vi "ROI entry-Previous ROI compat-Zoom.vi"(8 "error in (no error)":errorcluster, 9 "Proceed":bool=TRUE, 11 "Old ROI file path":path) -> (0 "error out":errorcluster, 1 "Proceed":bool, 3 "Old ROI file path (dup)":path)   [LabVIEW 2013]
uses:
  Visualisation/Functional Imaging Viewer/SubVIs/Experiment header interface/Typedefs/Header file type enum.ctl
  Visualisation/Functional Imaging Viewer/SubVIs/Experiment header interface/Typedefs/Save-Load-Save as-Load last enum.ctl
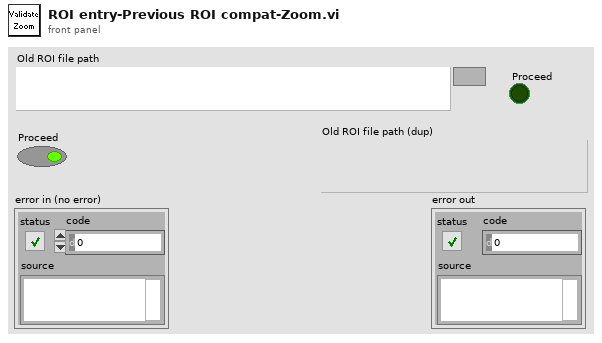
[diagram p1: front panel]
types:
  T1 = typedef "Save-Load-Save as-Load last enum.ctl" = enum16{"Save file", "Save file as", "Load file", "Load last file"}
  T2 = typedef "Header file type enum.ctl" = enum16{"All parameters", "Params for funct acq w ROI or mscn", "Params for funct acq w rectangles", "Live imaging header parameters", "AOL Parameters"}
  T3 = typedef "Fixed strings.ctl" = cluster{"ROI file name":string, "Normalised ROI file name":string, "Zplane Pockels values file name":string, "Functional data folder name":string, "Experiment Header file name":string, "Z-stack images folder name":string, "Groups setup rel. path":string, "Groups text file rel. path":string, "TDMS files folder name (F.img)":string, "TDMS files folder name (V.acq)":string, "TDMS files folder name (Pl.acq)":string, "Cycle rel times sequence file":string, "Dynamically called VIs folder name":string, "Time Series folder base name":string}
  T4 = typedef "Header parameters cluster-ALL.ctl" = cluster{"Imaging Protocol":T5, "Number of POI":u16, "Number of Miniscans":u16, "Number of Trials":u16, "Number of Cycles ":u64, "# Averaged Frames":u16, "Laser power (%)":u8, "Pockels":dbl, "Acquisition Length (sec)":dbl, "Fill time (us)":dbl, "POI Dwell time (us)":dbl, "Miniscan Dwell time per pixel (us)":dbl, "PMT 1":dbl, "PMT 2":dbl, "Back Apperture":dbl, "Zoom":dbl, "Frame Size":T6, "Center Frequency":dbl, "Field of View":dbl, "DwellTime (us)":dbl, "Wavelength (nm)":dbl, "AOL Z":dbl, "AOL Mode":T7, "GridXY":dbl, "GridZ":dbl, "TriggerDelay (sec)":dbl, "Number of Pixels in Miniscan":u16, "Experiment folder path":path, "X centre":dbl, "Y centre":dbl, "Angle (degrees)":dbl, "Plane Mode":T8, "Software version":dbl, "Objective":T9, "MotorZ Calibration":u32, "Pockels Calibration":u32, "Threshold":u16[], "Video length (sec)":dbl, "Frame rate (fps)":u8, "Rectangle ROI length (pixels)":u16, "Rectangle ROI height (pixels)":u16}
  T5 = typedef "Imaging Protocols enum.ctl" = enum16{"AOL Z-Stack", "Motor Z Stack", "Functional Acquisition", "Single Plane Acquisition", "Volume Acquisition", "Live Imaging", "Live Plane Imaging", "Live Volume Imaging"}
  T6 = typedef "Frame Size.ctl" = u16
  T7 = typedef "AOL modes.ctl" = enum16{"Raster", "Structural", "Pointing", "Mini Scan", "Alignment"}
  T8 = typedef "Plane Mode.ctl" = u16
  T9 = typedef "Objective selector control enum.ctl" = string
  T10 = typedef "AOL_Globals.ctl" = cluster{"Imaging Protocol":T5, "Number of POI":u16, "Number of Miniscans":u16, "Number of Trials":u16, "Number of Cycles ":u64, "# Averaged Frames":u16, "Laser power (%)":u8, "Pockels":dbl, "Acquisition Length (sec)":dbl, "Fill time (us)":dbl, "POI Dwell time (us)":dbl, "Miniscan Dwell time per pixel (us)":dbl, "PMT 1":dbl, "PMT 2":dbl, "Back Apperture":dbl, "Frame Size":T6, "Center Frequency":dbl, "Field of View":dbl, "DwellTime (us)":dbl, "Wavelength (nm)":dbl, "Zoom":dbl, "AOL Z":dbl, "AOL Mode":T7, "GridXY":dbl, "GridZ":dbl, "TriggerPeriod (sec)":dbl, "Number of Pixels in Miniscan":u16, "Experiment folder path":path, "X centre":dbl, "Y centre":dbl, "Angle (degrees)":dbl, "Plane Mode":T8, "Threshold":u16[], "Regenerate Chirps":bool, "Rectangle ROI length (pixels)":u16, "Rectangle ROI height (pixels)":u16, "AOD fill":u16, "Samples Wait after Trigger":u16, "StartUp Delay":i32, "Slip Cycle":u32, "Add Cycle":bool}
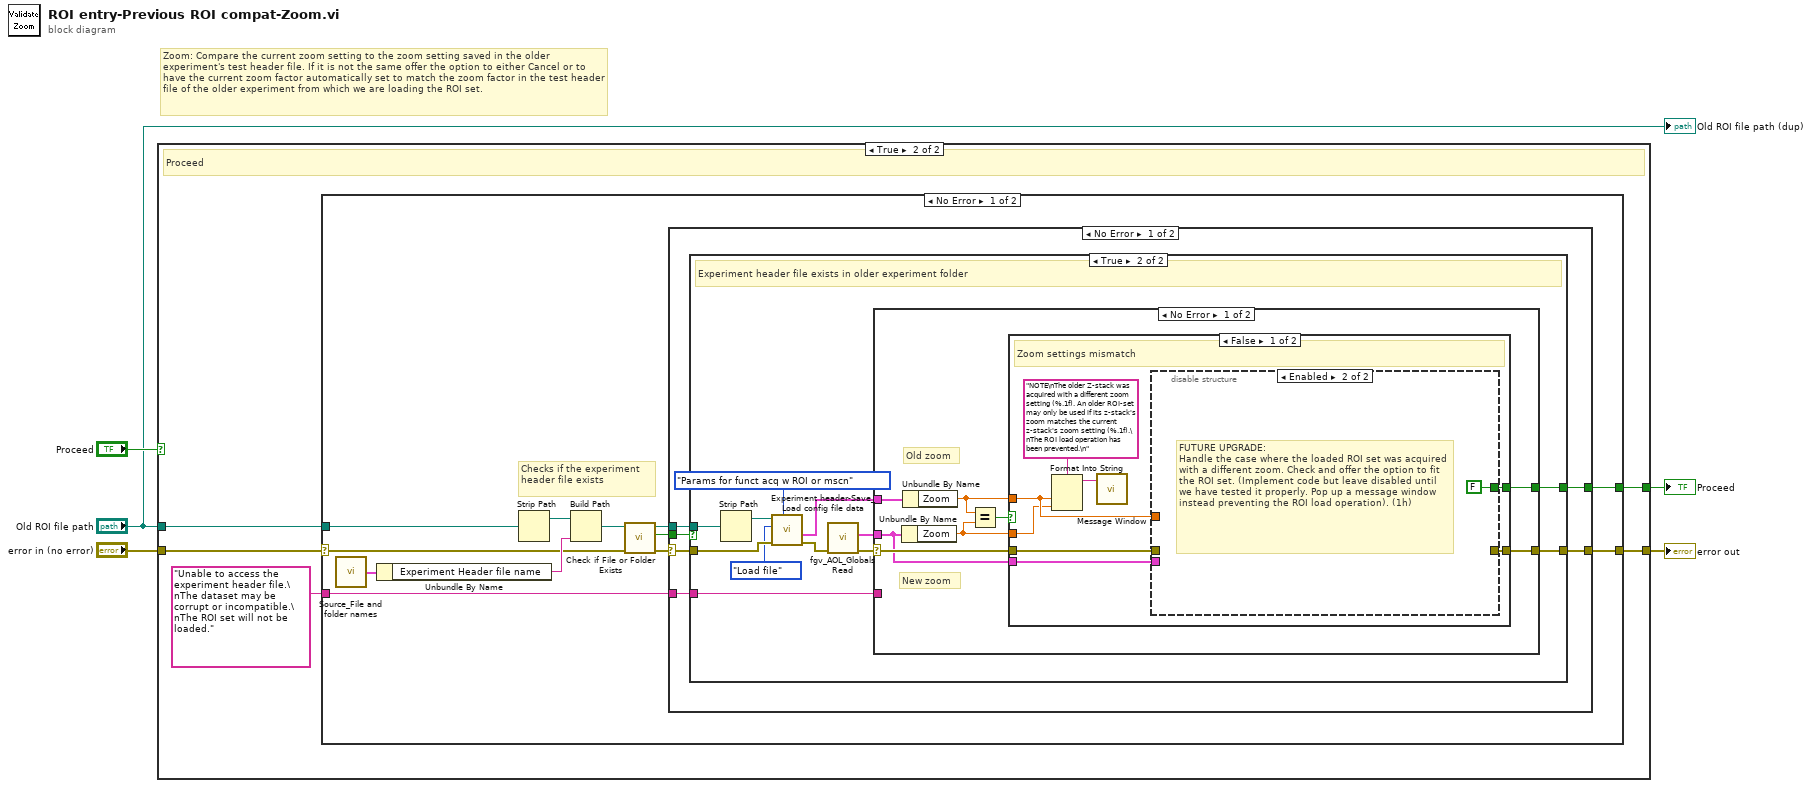
[diagram p0: block diagram]
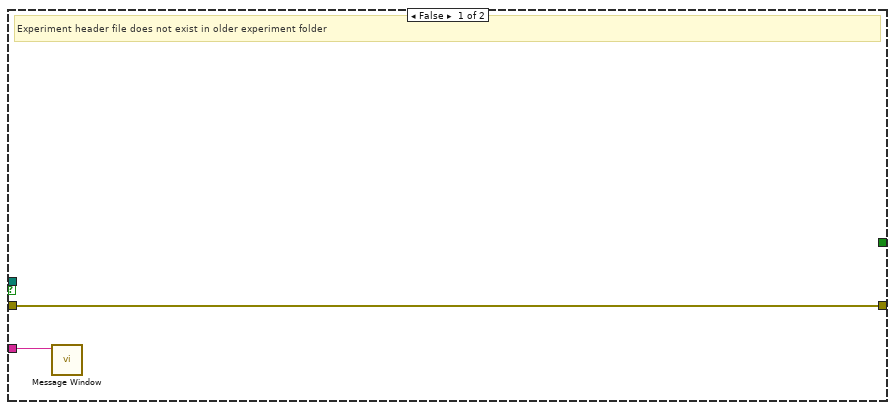
[diagram p3: hidden frame]
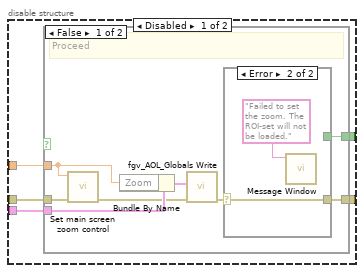
[diagram p4: hidden frame]
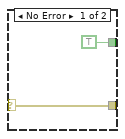
[diagram p5: hidden frame]
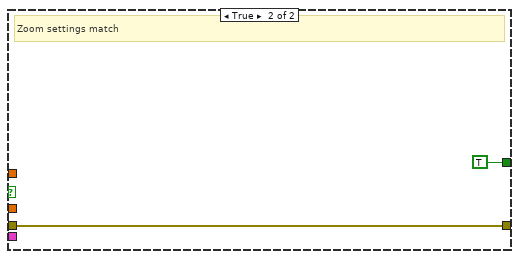
[diagram p7: hidden frame]
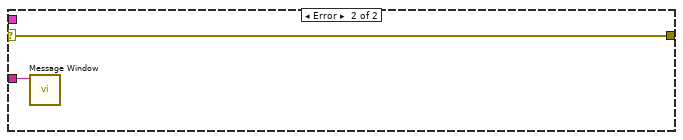
[diagram p8: hidden frame]
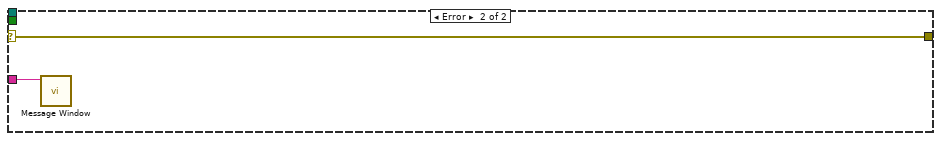
[diagram p9: hidden frame]
diagram:
  # "Zoom: Compare the current zoom setting to the zoom setting saved in the older experiment's test header file. If it is not the same offer the option to either Cancel or to have the current zoom factor automatically set to match the zoom factor in the test header file of the older experiment from which we are loading the ROI set."
  n1 = case shown="True" "Proceed" {
    tunnel: "Old ROI file path" -> [_ w11]
    tunnel: [w6 w9] -> w5
    tunnel: "error in (no error)" -> [w6 w8]
    tunnel: [_ w7] -> w3
    frame False {
      # "Skip"
    }
    frame True {
      # "Proceed"
      n2 = case shown="No Error" w8 {
        selector: w8 -> [w14 w85]
        tunnel: w11 -> [w21 _]
        tunnel: [w17 _] -> w7
        tunnel: [w13 w85] -> w9
        tunnel: "Unable to access the experiment header file.\nThe dataset may be corrupt or incompatible.\nThe ROI set will not be loaded." ("Message string") -> [w12 _]
        frame No Error {
          # "Checks if the experiment header file exists"
          n3 = call "Source_File and folder names.vi"() -> ("Fixed strings"=w22:T3)  [unwired: 1 in]
          n4 = Unbundle By Name(w22) -> ("Experiment Header file name"=w19:string)
          n5 = Strip Path(path=w21) -> (stripped path=w20:path)  [unwired: 1 out]
          n6 = Build Path(base path=w20, name or relative path=w19) -> (appended path=w23:path)
          n7 = call <vilib>:"Check if File or Folder Exists.vi"("error in (no error)"=w14, "path"=w23) -> ("error out"=w15:errorcluster, "file or folder exists?"=w18:bool, "dup path"=w16:path)  [unwired: 7 in]
          n8 = case shown="No Error" w15 {
            selector: w15 -> [w26 w84]
            tunnel: w18 -> [w29 _]
            tunnel: [w28 _] -> w17
            tunnel: w16 -> [w27 _]
            tunnel: [w25 w84] -> w13
            tunnel: w12 -> [w24 w83]
            frame No Error {
              n9 = case shown="True" w29 {
                tunnel: [_ w37] -> w28
                tunnel: w27 -> [_ w41]
                tunnel: w26 -> [w31 w39]
                tunnel: [w31 w36] -> w25
                tunnel: w24 -> [w30 w34]
                frame False {
                  # "Experiment header file does not exist in older experiment folder"
                  n10 = call "Message Window.vi"("Message string"=w30) -> ()  [unwired: 10 in, 1 out]
                }
                frame True {
                  # "Experiment header file exists in older experiment folder"
                  n11 = Strip Path(path=w41) -> (stripped path=w40:path)  [unwired: 1 out]
                  n12 = call "Experiment header-Save_Load config file data.vi"("Header file type"=Header_file_type_enum."Params for funct acq w ROI or mscn", "error in (no error)"=w39, "Function"=Save-Load-Save_as-Load_last_enum."Load file", "Experiment data folder path"=w40) -> ("error out"=w38:errorcluster, "All header parameters out"=w42:T4)  [unwired: 6 in]
                  n13 = call "fgv_AOL_Globals Read.vi"("error in (no error)"=w38) -> ("error out"=w35:errorcluster, "AOL_Globals"=w43:T10)  [unwired: 8 in, 1 out]
                  n14 = case shown="No Error" w35 {
                    selector: w35 -> [w47 w82]
                    tunnel: w43 -> [w45 _]
                    tunnel: w42 -> [w51 _]
                    tunnel: [w49 _] -> w37
                    tunnel: [w48 w82] -> w36
                    tunnel: w34 -> [_ w81]
                    frame No Error {
                      # "New zoom"
                      # "Old zoom"
                      n15 = Unbundle By Name(w45) -> ("Zoom"=w44:dbl)
                      n16 = Unbundle By Name(w51) -> ("Zoom"=w46:dbl)
                      n17 = Equal?(x=w46, y=w44) -> (x = y?=w50:bool)
                      n18 = case shown="False" w50 {
                        tunnel: [w59 TRUE] -> w49
                        tunnel: w47 -> [w57 w79]
                        tunnel: [w56 w79] -> w48
                        tunnel: w46 -> [w58 _]
                        tunnel: w45 -> [w55 _]
                        tunnel: w44 -> [w53 _]
                        frame False {
                          # "Zoom settings mismatch"
                          n19 = Format Into String(format string="NOTE\nThe older Z-stack was acquired with a different zoom setting (%.1f). An older ROI-set may only be used if its z-stack's zoom matches the current z-stack's zoom setting (%.1f).\nThe ROI load operation has been prevented.\n" ("Message string"), w58, w53) -> (resulting string=w52:string)  [unwired: 2 in, 1 out]
                          n20 = call "Message Window.vi"("Message string"=w52) -> ()  [unwired: 10 in, 1 out]
                          n21 = disable-structure shown="Enabled" {
                            disable-tunnel: [w64 FALSE] -> w59
                            disable-tunnel: w58 -> [w63 _]
                            disable-tunnel: w57 -> [w62 _]
                            disable-tunnel: [w61 _] -> w56
                            disable-tunnel: w55 -> [w60 _]
                            frame Disabled {
                              n22 = case shown="False" {
                                selector: _ -> [_ _]
                                tunnel: [w72 _] -> w64
                                tunnel: w63 -> [w69 _]
                                tunnel: w62 -> [w68 w77]
                                tunnel: [w65 w77] -> w61
                                tunnel: w60 -> [w71 _]
                                frame False {
                                # "Proceed"
                                n23 = call "Set main screen zoom control.vi"("error in (no error)"=w68, "Zoom"=w69) -> ("error out"=w67:errorcluster)  [unwired: 9 in]
                                n24 = Bundle By Name(cluster=w71, "Zoom"=w69) -> (w70:T10)
                                n25 = call "fgv_AOL_Globals Write.vi"("error in (no error)"=w67, "AOL_Globals"=w70) -> ("error out"=w66:errorcluster)  [unwired: 9 in]
                                n26 = case shown="Error" w66 {
                                selector: w66 -> [w73 w76]
                                tunnel: [TRUE _] -> w72
                                tunnel: [w73 w76] -> w65
                                frame No Error {
                                }
                                frame Error {
                                n27 = call "Message Window.vi"("Message string"="Failed to set the zoom. The ROI-set will not be loaded.") -> ()  [unwired: 10 in, 1 out]
                                }
                                }
                                }
                                frame True {
                                # "Cancelled"
                                }
                              }
                            }
                            frame Enabled {
                              # "FUTURE UPGRADE:\nHandle the case where the loaded ROI set was acquired with a different zoom. Check and offer the option to fit the ROI set. (Implement code but leave disabled until we have tested it properly. Pop up a message window instead preventing the ROI load operation). (1h)"
                            }
                          }
                        }
                        frame True {
                          # "Zoom settings match"
                        }
                      }
                    }
                    frame Error {
                      n28 = call "Message Window.vi"("Message string"=w81) -> ()  [unwired: 10 in, 1 out]
                    }
                  }
                }
              }
            }
            frame Error {
              n29 = call "Message Window.vi"("Message string"=w83) -> ()  [unwired: 10 in, 1 out]
            }
          }
        }
        frame Error {
        }
      }
    }
  }
  "error out" <- w5
  "Proceed" <- w3
  "Old ROI file path (dup)" <- "Old ROI file path"
